vi "Disconnect.vi"(8 "error in":errorcluster, 11 "6700 in":refnum<class "6700.lvclass">) -> (0 "error out":errorcluster, 3 "6700 out":refnum<class "6700.lvclass">)   [LabVIEW 2018, in "6700.lvlib" / "6700.lvclass"]
uses:
  6700.lvclass
  <instrlib>/Agilent N6700 Series/Agilent N6700 Series.lvlib
  builds/Power_Supply.lvlibp/Power Supply.lvclass
  C:/Users/Ron.Dexter.LUMINARTECH/Desktop/builds/Power_Supply.lvlibp/Power Supply.lvclass
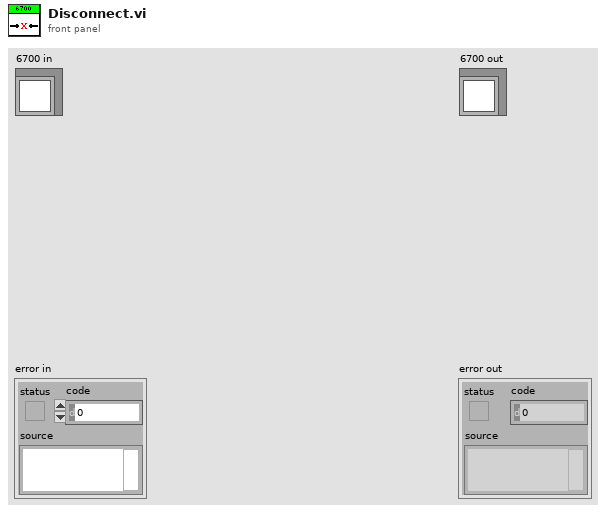
[diagram p1: front panel]
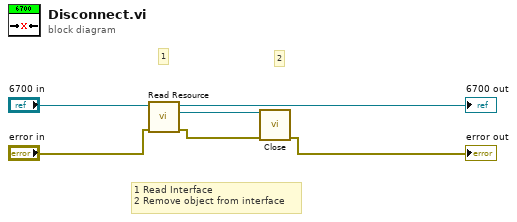
[diagram p0: block diagram]
diagram:
  # "1 Read Interface\n2 Remove object from interface"
  # "2"
  # "1"
  n1 = call "Read Resource.vi"("error in"="error in", "Power Supply in"="6700 in") -> ("error out"=w3:errorcluster, "Resource"=w4:refnum<visa-resource-name>, "Power Supply out"=→"6700 out":refnum<class "6700.lvclass">)  [unwired: 7 in]
  n2 = call <instrlib>:"Close.vi"("VISA resource name"=w4, "error in (no error)"=w3) -> ("error out"=→"error out":errorcluster)  [unwired: 13 in]
